vi "加标回收率计算.vi"(11 "参数":T1) -> (3 "参数 out":T1)   [LabVIEW 2016, in "质控单元.lvlib"]
panel:
  out "V1":dbl
  out "R":dbl
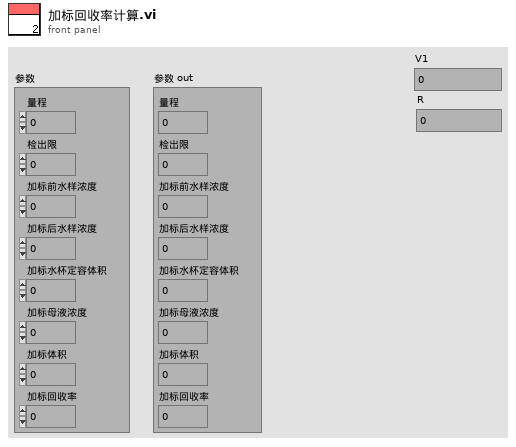
[diagram p1: front panel]
types:
  T1 = cluster{"量程":dbl, "检出限":dbl, "加标前水样浓度":dbl, "加标后水样浓度":dbl, "加标水杯定容体积":dbl, "加标母液浓度":dbl, "加标体积":dbl, "加标回收率":dbl}
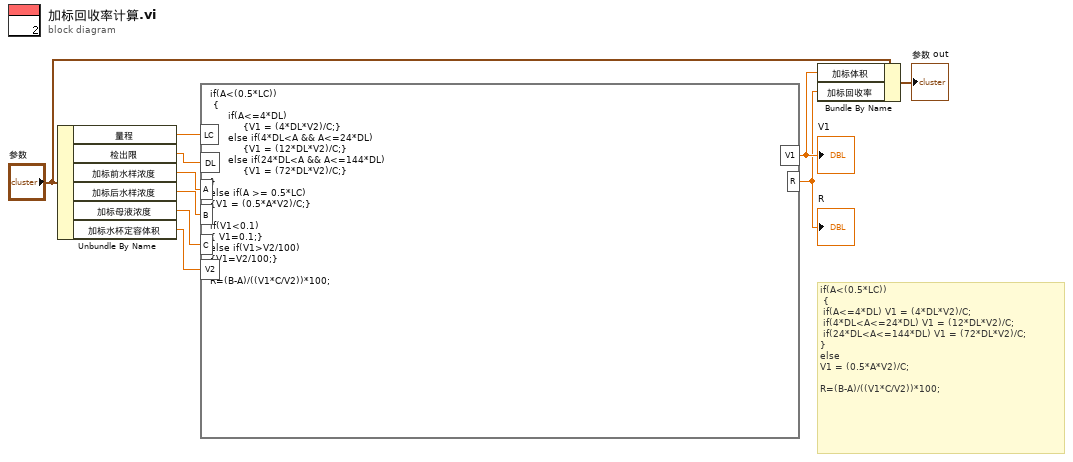
[diagram p0: block diagram]
diagram:
  # "if(A<(0.5*LC))\n {\n if(A<=4*DL) V1 = (4*DL*V2)/C;\n if(4*DL<A<=24*DL) V1 = (12*DL*V2)/C;\n if(24*DL<A<=144*DL) V1 = (72*DL*V2)/C;\n}\nelse\nV1 = (0.5*A*V2)/C;\n\nR=(B-A)/((V1*C/V2))*100;"
  n1 = Unbundle By Name("参数") -> ("量程"=w7:dbl, "检出限"=w6:dbl, "加标前水样浓度"=w10:dbl, "加标后水样浓度"=w9:dbl, "加标母液浓度"=w8:dbl, "加标水杯定容体积"=w5:dbl)
  n2 = formula code="if(A<(0.5*LC))\n {\n      if(A<=4*DL) \n           {V1 = (4*DL*V2)/C;}\n      else if(4*DL<A && A<=24*DL) \n           {V1 = (12*DL*V2)/C;}\n      else if(24*DL<A && A<=144*DL) \n           {V1 = (72*DL*V2)/C;}\n}\nelse if(A >= 0.5*LC)\n{V1 = (0.5*A*V2)/C;}\n\nif(V1<0.1)\n{ V1=0.1;}\nelse if(V1>V2/100)\n{V1=V2/100;}\n\nR=(B-A)/((V1*C/V2))*100;"("A"=w10, "B"=w9, "C"=w8, "V2"=w5, "LC"=w7, "DL"=w6) -> ("R"=w2:dbl, "V1"=w3:dbl)
  "R" <- w2
  "V1" <- w3
  n3 = Bundle By Name(cluster="参数", "加标体积"=w3, "加标回收率"=w2) -> (→"参数 out":T1)
